vi "writeframedata.vi"(6 "trigger number":dbl, 8 "pathname":path, 9 "data frames / trigger":dbl, 10 "video frames / data frame":dbl, 11 "Images In":T1[](array[typedef])) -> ()   [LabVIEW 2009]
uses:
  <vilib>/vision/Image Controls.llb/IMAQ Image.ctl
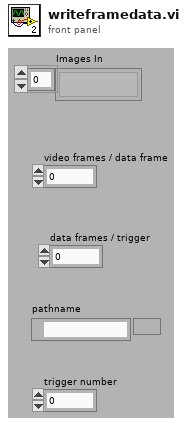
[diagram p1: front panel]
types:
  T1 = typedef "IMAQ Image.ctl" = refnum<image>
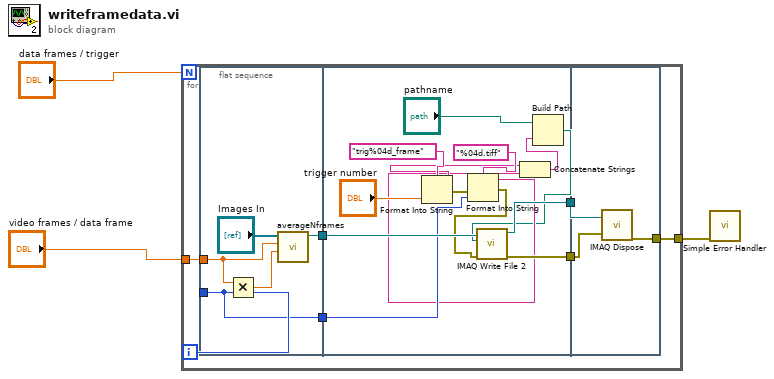
[diagram p0: block diagram]
diagram:
  n1 = for {
    N: "data frames / trigger" -> [_]
    tunnel: [w7] -> w3
    tunnel: "video frames / data frame" -> [w6]
    i -> [w5]
    n2 = flat-sequence {
      tunnel: [w15] -> w10
      tunnel: w6 -> [w13]
      tunnel: w5 -> [w11]
      tunnel: [w11] -> w4
      tunnel: w10 -> [w29]
      tunnel: [w28] -> w9
      tunnel: [w27] -> w8
      tunnel: w4 -> [w21]
      tunnel: w9 -> [w32]
      tunnel: w8 -> [w31]
      tunnel: [w30] -> w7
      frame #0 {
        n3 = Multiply(x=w13, y=w11) -> (x*y=w12:dbl)
        n4 = call "averageNframes.vi"("first frame index"=w12, "number of frames"=w13, "Images In"="Images In") -> ("Image out"=w15:T1)  [unwired: 8 in]
      }
      frame #1 {
        n5 = Format Into String(format string="trig%04d_frame", "trigger number") -> (resulting string=w19:string, error out=w23:errorcluster)  [unwired: 2 in]
        n6 = Format Into String(format string="%04d.tiff", error in=w23, w21) -> (resulting string=w18:string, error out=w22:errorcluster)  [unwired: 1 in]
        n7 = Concatenate Strings(w19, w18) -> (w17:string)
        n8 = Build Path(base path="pathname", name or relative path=w17) -> (appended path=w16:path)
        n9 = call-poly "IMAQ Write File 2"("error in (no error)"=w22, "File Path"=w16, "Image"=w29) -> ("error out"=w27:errorcluster, "Image Out (duplicate)"=w28:T1)  [unwired: 7 in]
      }
      frame #2 {
        n10 = call "IMAQ Dispose"("Image"=w32, "error in (no error)"=w31) -> ("error out"=w30:errorcluster)  [unwired: 4 in]
      }
    }
  }
  n11 = call <vilib>:"Simple Error Handler.vi"("error in (no error)"=w3) -> ()  [unwired: 4 in, 5 out]
